vi "mmWaveTesterFilePaths.vi"() -> (0 "error out":errorcluster, 1 "Data Files Dir":path, 2 "Config File Path Motion":path, 3 "Config File Path":path, 5 "exe?":bool, 6 "Public Preferences":path)   [LabVIEW 2019]
doc: "Defines directories where the XRTC config files go.\nIf the directories aren't there executing this VI creates them.\nThe absolute path for each directory may be different on windows XP and Win7"
uses:
  <vilib>/Utility/sysdir.llb/System Directory Type.ctl
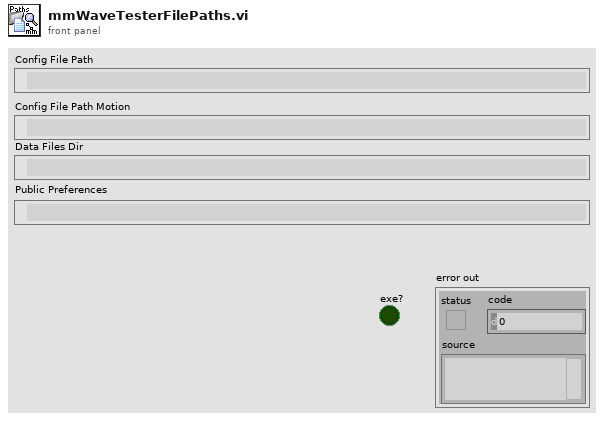
[diagram p1: front panel]
types:
  T1 = enum32{"invalid app kind", "Development System", "Run Time System", "Student Edition", "Embedded LabVIEW", "Evaluation", "Custom"}
  T2 = typedef "System Directory Type.ctl" = i32
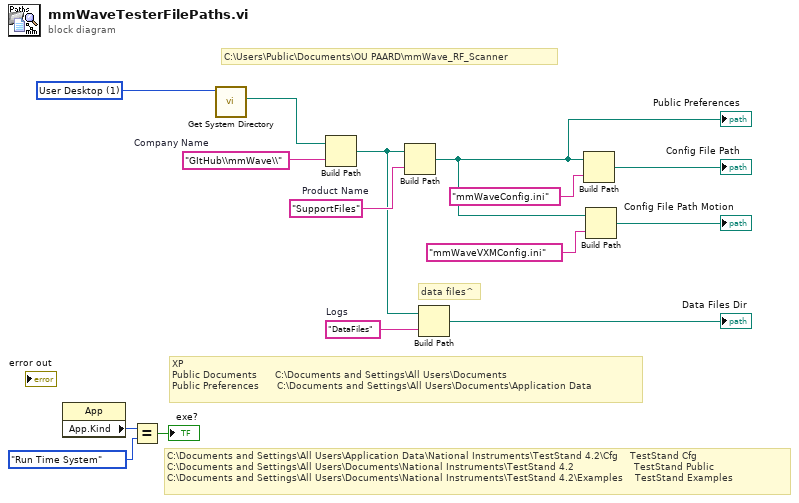
[diagram p0: block diagram]
diagram:
  w10 = "DataFiles"  # Logs
  w13 = "SupportFiles"  # Product Name
  w12 = "GItHub\\mmWave\\"  # Company Name
  w15 = T2 1 items=["User Home", "User Desktop", "User Documents", "User Application Data", "User Preferences", "User Temporary", "Public Documents", "Public Application Data", "Public Preferences", "System Core Libraries", "System Installed Libraries", "Application Files", "Boot Volume Root"] ("system directory type")
  # "C:\\Users\\Public\\Documents\\OU PAARD\\mmWave_RF_Scanner"
  # "XP\nPublic Documents      C:\\Documents and Settings\\All Users\\Documents\nPublic Preferences      C:\\Documents and Settings\\All Users\\Documents\\Application Data"
  # "C:\\Documents and Settings\\All Users\\Application Data\\National Instruments\\TestStand 4.2\\Cfg\t   TestStand Cfg\nC:\\Documents and Settings\\All Users\\Documents\\National Instruments\\TestStand 4.2\t                   TestStand Public\nC:\\Documents and Settings\\All Users\\Documents\\National Instruments\\TestStand 4.2\\Examples\t   TestStand Examples"
  # "data files^"
  n1 = property class="App"() -> ("App.Kind"=w7:T1)  [unwired: 2 in, 2 out]
  n2 = Equal?(x=w7, y=T1."Run Time System" ("Application:Kind")) -> (x = y?=→"exe?":bool)
  n3 = call <vilib>:"Get System Directory.vi"("system directory type"=w15) -> ("system directory"=w14:path)  [unwired: 10 in]
  n4 = Build Path(base path=w14, name or relative path=w12) -> (appended path=w5:path)
  n5 = Build Path(base path=w5, name or relative path=w13) -> (appended path=w1:path)
  "Public Preferences" <- w1
  n6 = Build Path(base path=w5, name or relative path=w10) -> (appended path=→"Data Files Dir":path)
  n7 = Build Path(base path=w1, name or relative path="mmWaveConfig.ini") -> (appended path=→"Config File Path":path)
  n8 = Build Path(base path=w1, name or relative path="mmWaveVXMConfig.ini") -> (appended path=→"Config File Path Motion":path)
